vi "Rel.vi"(0 "VisaCluster":T1, 7 "Rel":bool, 11 "error in (no error)":errorcluster) -> (4 "VisaCluster":T1, 6 "Boolean":bool=TRUE, 8 "Answer":string, 10 "Display":string, 15 "error out":errorcluster)   [LabVIEW 2014, in "FH 55.lvlib"]
doc: "This VI sets the Relative ON or OFF. \n\nDas VI Rel wird zum Ein- bzw. Ausschalten der Relativ-Funktion verwendet. Mit der Funktion Relative können kleine Änderungen in großen Magnetfeldern leichter beobachtet werden. Ist die Funktion eingeschaltet, werden nur die Abweichungen von einem zuvor gewählten Bezugswert angezeigt."
uses:
  FH 55.lvlib
  TypeDef/VisaCluster.ctl
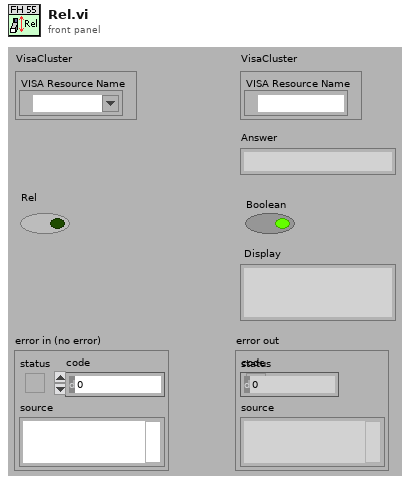
[diagram p1: front panel]
types:
  T1 = typedef "FH 55.lvlib/VisaCluster.ctl" = cluster{"VISA Resource Name":refnum<visa-resource-name>}
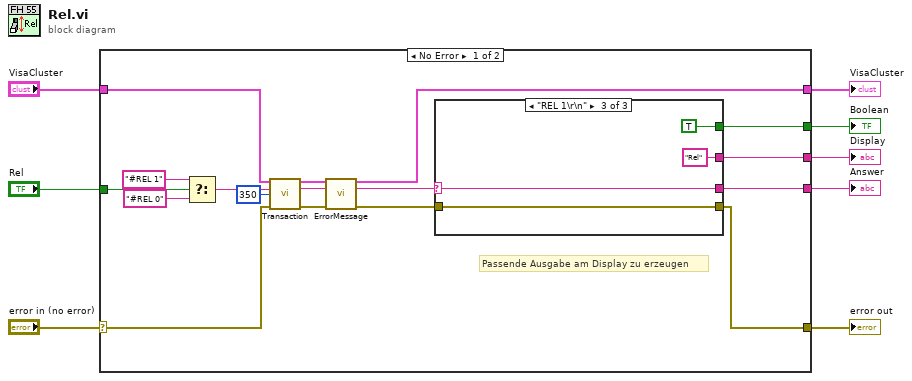
[diagram p0: block diagram]
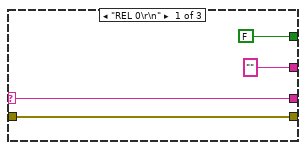
[diagram p2: hidden frame]
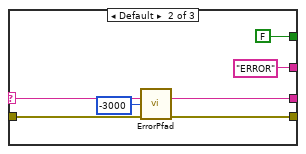
[diagram p3: hidden frame]
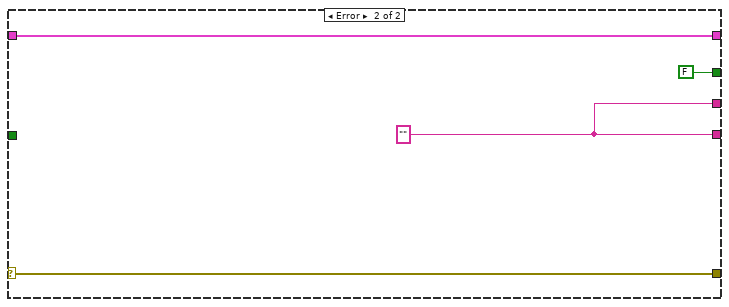
[diagram p4: hidden frame]
diagram:
  n1 = case shown="No Error" "error in (no error)" {
    selector: "error in (no error)" -> [w20 w42]
    tunnel: "VisaCluster" -> [w22 w43]
    tunnel: "Rel" -> [w25 _]
    tunnel: [w16 w43] -> w4
    tunnel: [w10 w42] -> w6
    tunnel: [w17 w41] -> w5
    tunnel: [w15 w41] -> w2
    tunnel: [w9 FALSE] -> w1
    frame No Error {
      # "Passende Ausgabe am Display zu erzeugen"
      n2 = Select(t="#REL 1", s=w25, f="#REL 0") -> (s? t:f=w21:string)
      n3 = call "Transaction.vi"("VisaCluster"=w22, "Command"=w21, "Time (150) ms"=u32 350, "error in (no error)"=w20) -> ("VisaCluster"=w13:T1, "Answer"=w19:string, "error out"=w12:errorcluster)  [unwired: 8 in, 1 out]
      n4 = call "ErrorMessage.vi"("VisaCluster"=w13, "Message In"=w19, "error in (no error)"=w12) -> ("VisaCluster"=w16:T1, "Message Out"=w18:string, "error out"=w11:errorcluster)  [unwired: 10 in]
      n5 = case shown="\"REL 1\\r\\n\"" w18 {
        selector: w18 -> [w29 w31 w39]
        tunnel: [w29 w31 w39] -> w17
        tunnel: ["" "ERROR" "Rel"] -> w15
        tunnel: w11 -> [w27 w32 w38]
        tunnel: [w27 w35 w38] -> w10
        tunnel: [FALSE FALSE TRUE] -> w9
        frame "REL 0\r\n" {
        }
        frame Default {
          n6 = call "ErrorPfad.vi"("Message In"=w31, "Numeric"=-3000 ("code"), "error in (no error)"=w32) -> ("error out"=w35:errorcluster)  [unwired: 11 in, 1 out]
        }
        frame "REL 1\r\n" {
        }
      }
    }
    frame Error {
      w41 = ""
    }
  }
  "error out" <- w6
  "Answer" <- w5
  "VisaCluster" <- w4
  "Display" <- w2
  "Boolean" <- w1
